vi "Handle Error.vi"(8 "error in (no error)":errorcluster, 11 "Application in":refnum<class "Application.lvclass">) -> (0 "error out":errorcluster, 2 "stop actor?":bool=TRUE, 3 "Application out":refnum<class "Application.lvclass">)   [LabVIEW 2018, in "Application.lvlib" / "Application.lvclass"]
doc: "(<B>Filename</B>: Actor Framework.lvlib:Actor.lvclass:Handle Error.vi)\n\nDefines how the actor handles an error that occurred while processing a message. By default, this method does nothing except stop the actor."
uses:
  Application.lvclass
  <vilib>/ActorFramework/Actor/Actor.lvclass
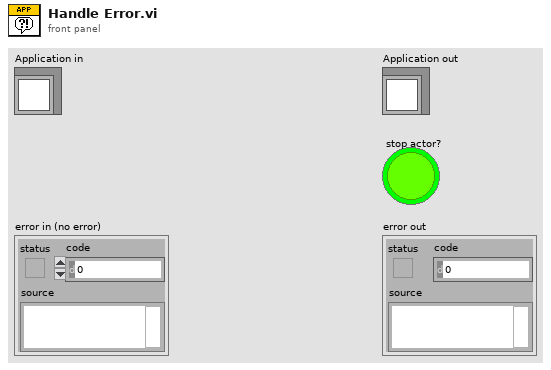
[diagram p1: front panel]
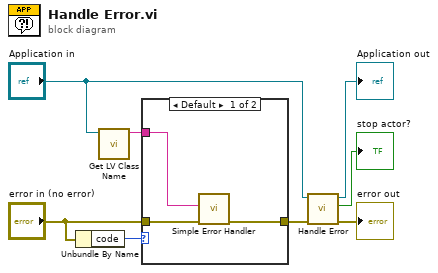
[diagram p0: block diagram]
diagram:
  n1 = Unbundle By Name("error in (no error)") -> ("code"=w1:i32)
  n2 = call <vilib>:"Get LV Class Name.vi"("object"="Application in") -> ("class name"=w3:string)  [unwired: 9 in, 1 out]
  n3 = case shown="Default" w1 {
    tunnel: [w11 w12] -> w5
    tunnel: w3 -> [w10 _]
    tunnel: "error in (no error)" -> [w9 w12]
    frame Default {
      n4 = call <vilib>:"Simple Error Handler.vi"("error source (\" \")"=w10, "error in (no error)"=w9) -> ("error out"=w11:errorcluster)  [unwired: 3 in, 4 out]
    }
    frame 0, 43, 1608 {
    }
  }
  n5 = call-parent "Handle Error.vi"("error in (no error)"=w5, "Actor in"="Application in") -> ("error out"=→"error out":errorcluster, "stop actor?"=→"stop actor?":bool, "Actor out"=→"Application out":refnum<class "Application.lvclass">)  [unwired: 7 in]
